vi "Create Message Queue Reference.vi"(8 "error in (no error)":errorcluster) -> (0 "error out":errorcluster)   [LabVIEW 2021, in "dcvmMessageQueue.lvlib"]
uses:
  dcvmMessageQueue.lvlib
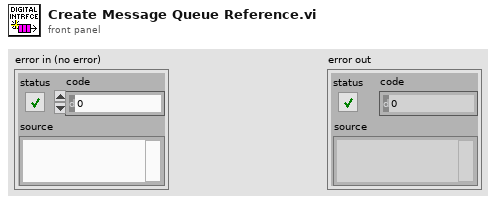
[diagram p1: front panel]
types:
  T1 = typedef "dcvmMessageQueue.lvlib/Message Queues.ctl" = cluster{"gRPC engine":refnum<queue>, "Digital engine":refnum<queue>}
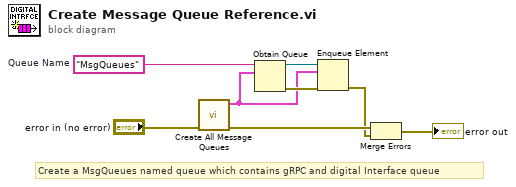
[diagram p0: block diagram]
diagram:
  w1 = "MsgQueues"  # Queue Name
  # "Create a MsgQueues named queue which contains gRPC and digital Interface queue"
  n1 = call "Create All Message Queues.vi"("error in (no error)"="error in (no error)") -> ("error out"=w5:errorcluster, "Message queues out"=w2:T1)  [unwired: 9 in]
  n2 = Obtain Queue(name (unnamed)=w1, element data type=w2) -> (queue out=w7:refnum<queue>, error out=w6:errorcluster)  [unwired: 3 in, 1 out]
  n3 = Enqueue Element(queue=w7, element=w2, error in (no error)=w6) -> (error out=w4:errorcluster)  [unwired: 1 in, 2 out]
  n4 = Merge Errors(w5, w4) -> (→"error out":errorcluster)
